vi "Create-romi-sim-model.vi"() -> (2 "Encoder Ft/Count":dbl, 3 "out DiffDriveTrainSim":T1 {"m_Motor"."Jr_KgM2" format="%13.5p"; "m_Motor"."L_H" format="%13.5p"; "m_Motor"."Kt_NMPerAmp" format="%13.5p"; "m_Motor"."KvINV_RadPerSecPerVolt" format="%13.5p"; "m_Motor"."R_Ohms" format="%13.5p"; "m_Motor"."FreeSpeed_RadPerSec" format="%13.5p"; "m_Motor"."FreeCurrent_Amps" format="%13.5p"; "m_Motor"."StallCurrent_Amps" format="%13.5p"; "m_Motor"."StallTorque_NM" format="%13.5p"; "m_Motor"."nominalVoltage_Volts" format="%13.5p"})   [LabVIEW 2020]
uses:
  <vilib>/Rock Robotics/WPI/ThirdParty/JAS_Junk/TrajLib/DIFF_DRIVE_TRAIN_SIM.ctl
  <vilib>/Rock Robotics/WPI/ThirdParty/JAS_Junk/TrajLib/LINEAR_SYSTEM.ctl
  <vilib>/Analysis/Matrix/Datatypes/RealMatrix.ctl
  <vilib>/Rock Robotics/WPI/ThirdParty/JAS_Junk/TrajLib/DCMOTOR.CTL
  <vilib>/Rock Robotics/WPI/ThirdParty/JAS_Junk/TrajLib/DCMOTOR_TYPES_ENUM.ctl
  <vilib>/Rock Robotics/WPI/ThirdParty/JAS_Junk/TrajLib/DCMotor_GetCIM.vi
  <vilib>/Rock Robotics/WPI/ThirdParty/JAS_Junk/TrajLib/DCMotor_GetAndymark9015.vi
  <vilib>/Rock Robotics/WPI/ThirdParty/JAS_Junk/TrajLib/DCMotor_GetAndymarkRs775_125.vi
  <vilib>/Rock Robotics/WPI/ThirdParty/JAS_Junk/TrajLib/DCMotor_GetBag.vi
  <vilib>/Rock Robotics/WPI/ThirdParty/JAS_Junk/TrajLib/DCMotor_GetBanebotsRs550.vi
  <vilib>/Rock Robotics/WPI/ThirdParty/JAS_Junk/TrajLib/DCMotor_GetBanebotsRs775.vi
  <vilib>/Rock Robotics/WPI/ThirdParty/JAS_Junk/TrajLib/DCMotor_GetFalcon500.vi
  <vilib>/Rock Robotics/WPI/ThirdParty/JAS_Junk/TrajLib/DCMotor_GetMiniCIM.vi
  <vilib>/Rock Robotics/WPI/ThirdParty/JAS_Junk/TrajLib/DCMotor_GetNEO.vi
  <vilib>/Rock Robotics/WPI/ThirdParty/JAS_Junk/TrajLib/DCMotor_GetNEO550.vi
  <vilib>/Rock Robotics/WPI/ThirdParty/JAS_Junk/TrajLib/DCMotor_GetRomiBuiltIn.vi
  <vilib>/Rock Robotics/WPI/ThirdParty/JAS_Junk/TrajLib/DCMotor_GetVex775Pro.vi
  <vilib>/Rock Robotics/WPI/ThirdParty/JAS_Junk/TrajLib/LinearSystem_New.vi
  <vilib>/Rock Robotics/WPI/ThirdParty/JAS_Junk/TrajLib/MatBuilder_Create.vi
  <vilib>/Rock Robotics/WPI/ThirdParty/JAS_Junk/TrajLib/MatBuilder_Fill.vi
  <vilib>/Rock Robotics/WPI/ThirdParty/JAS_Junk/TrajLib/MatrixHelper_Zero.vi
  <vilib>/Rock Robotics/WPI/ThirdParty/JAS_Junk/TrajLib/Rotation_CreateAngle.vi
  <vilib>/Rock Robotics/WPI/ThirdParty/JAS_Junk/TrajLib/Translation_Create.vi
  <vilib>/Rock Robotics/WPI/ThirdParty/JAS_Junk/TrajLib/DCMotor_New.vi
  <vilib>/Rock Robotics/WPI/ThirdParty/JAS_Junk/TrajLib/Units_RotationsPerMinuteToRadiansPerSecond.vi
  <vilib>/Rock Robotics/WPI/ThirdParty/JAS_Junk/TrajLib/MatrixHelper_CoerceSize.vi
  <vilib>/Rock Robotics/WPI/ThirdParty/JAS_Junk/TrajLib/Trajectory_Library.lvlib
  <vilib>/Analysis/Matrix/NI_Matrix.lvlib
panel:
  # "<States, 1>"
  # "<Outputs, 1>"
  # "<Inputs, 1>"
  # "<Outputs, 1>"
  # "<States,States>"
  # "<States,Inputs>"
  # "<Outputs,States>"
  # "<Outputs,Inputs>"
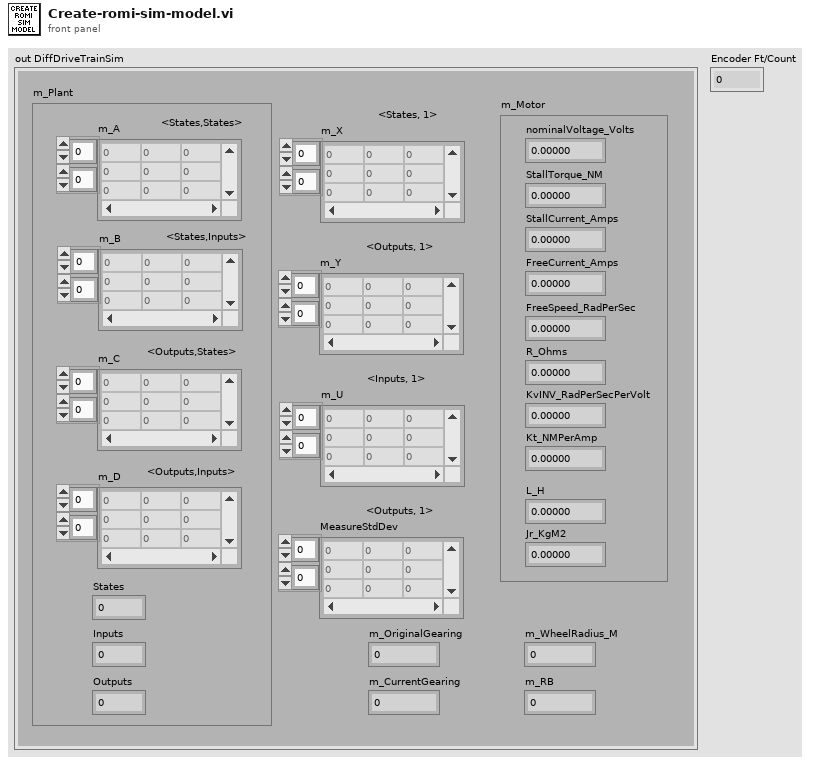
[diagram p1: front panel]
types:
  T1 = typedef "Trajectory_Library.lvlib/DIFF_DRIVE_TRAIN_SIM.ctl" = cluster{"m_Plant":T2, "m_X":T3, "m_Y":T3, "m_U":T3, "MeasureStdDev":T3, "m_Motor":T4, "m_OriginalGearing":dbl, "m_CurrentGearing":dbl, "m_WheelRadius_M":dbl, "m_RB":dbl}
  T2 = typedef "Trajectory_Library.lvlib/LINEAR_SYSTEM.ctl" = cluster{"m_A":T3, "m_B":T3, "m_C":T3, "m_D":T3, "States":i32, "Inputs":i32, "Outputs":i32}
  T3 = typedef "NI_Matrix.lvlib/RealMatrix.ctl" = dbl[][]
  T4 = typedef "Trajectory_Library.lvlib/DCMOTOR.CTL" = cluster{"nominalVoltage_Volts":dbl, "StallTorque_NM":dbl, "StallCurrent_Amps":dbl, "FreeCurrent_Amps":dbl, "FreeSpeed_RadPerSec":dbl, "R_Ohms":dbl, "KvINV_RadPerSecPerVolt":dbl, "Kt_NMPerAmp":dbl, "L_H":dbl, "Jr_KgM2":dbl}
  T5 = typedef "Trajectory_Library.lvlib/DCMOTOR_TYPES_ENUM.ctl" = enum16{"CIM", "AndyMark 9015", "Andy Mark RS 775 125", "Bag", "BaneBots RS 550", "BaneBots RS 775", "Falcon 500", "Mini CIM", "NEO", "NEO 550", "Romi BuiltIn", "Vex 775 Pro"}
  T6 = typedef "Trajectory_Library.lvlib/POSE2D.ctl" = cluster{"TRANSLATION":T7, "ROTATION":T8}
  T7 = typedef "Trajectory_Library.lvlib/TRANSLATION2D.ctl" = cluster{"X":dbl, "Y":dbl}
  T8 = typedef "Trajectory_Library.lvlib/ROTATION2D.ctl" = cluster{"VALUE":dbl, "COS":dbl, "SIN":dbl}
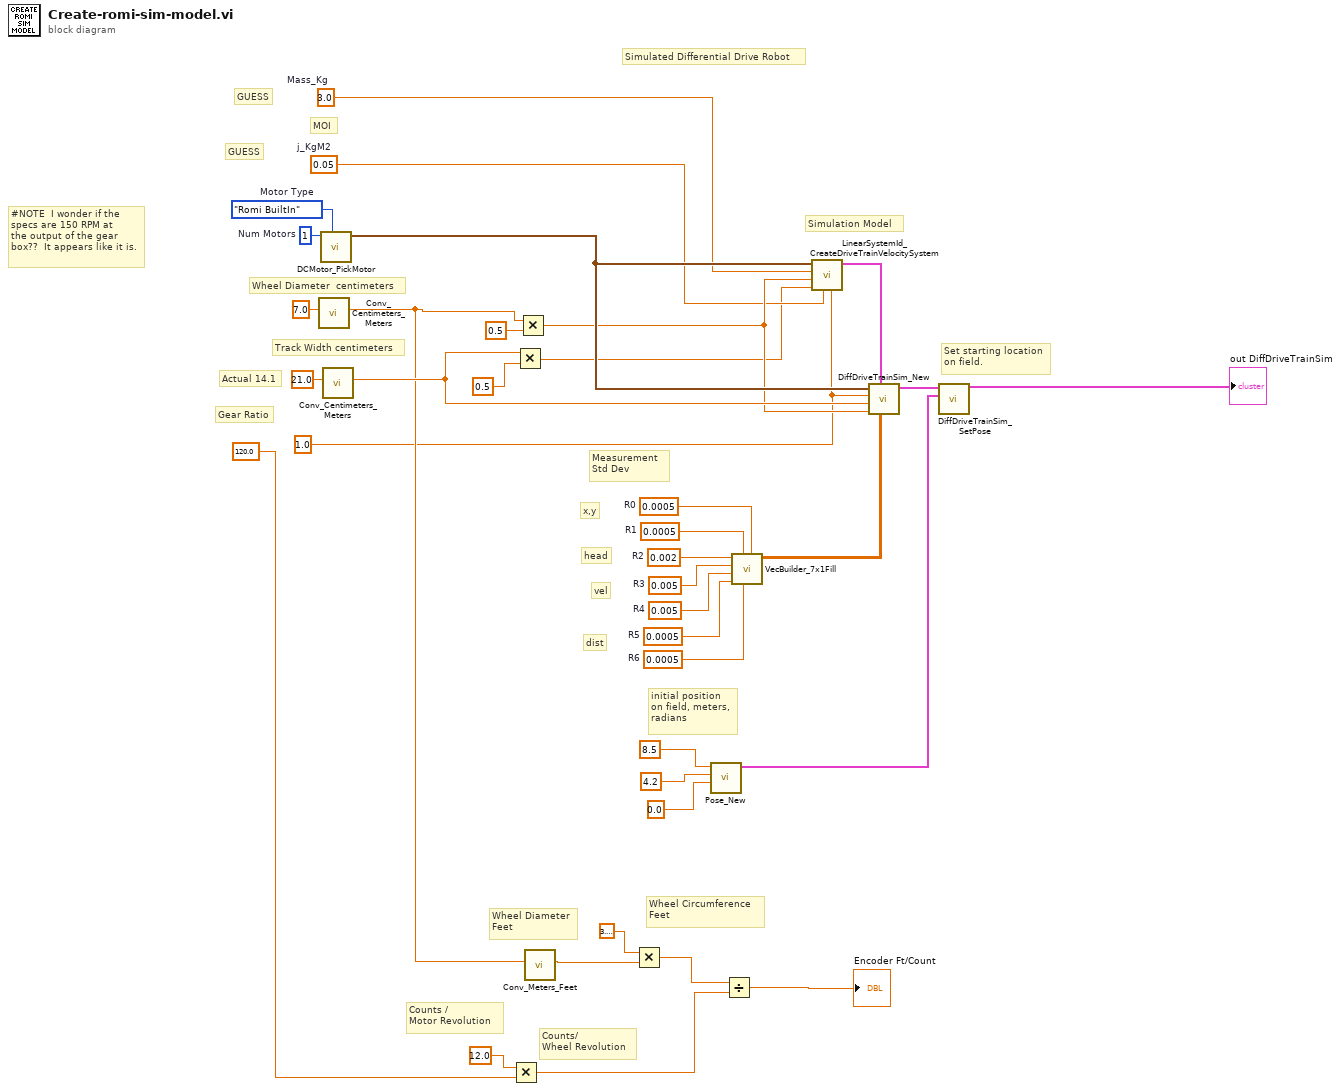
[diagram p0: block diagram]
diagram:
  w1 = 1.0 ("INCH")
  w30 = 1  # Num Motors
  w31 = DCMOTOR_TYPES_ENUM."Romi BuiltIn"  # Motor Type
  w24 = 3.0  # Mass_Kg
  w26 = 0.05  # j_KgM2
  w15 = 0.0005  # R6
  w16 = 0.0005  # R5
  w17 = 0.005  # R4
  w18 = 0.005  # R3
  w19 = 0.002  # R2
  w20 = 0.0005  # R1
  w21 = 0.0005  # R0
  # "Actual 14.1"
  # "#NOTE  I wonder if the \nspecs are 150 RPM at\nthe output of the gear\nbox??  It appears like it is."
  # "Wheel Circumference\nFeet"
  # "Wheel Diameter\nFeet"
  # "Counts/\nWheel Revolution"
  # "Counts /\nMotor Revolution"
  # "Set starting location\non field."
  # "Measurement \nStd Dev"
  # "Gear Ratio"
  # "GUESS"
  # "GUESS"
  # "Track Width centimeters"
  # "Wheel Diameter  centimeters"
  # "MOI"
  # "dist"
  # "vel"
  # "head"
  # "x,y"
  # "Simulated Differential Drive Robot"
  # "initial position\non field, meters,\nradians"
  # "Simulation Model"
  n1 = call <vilib>:"Conv_Centimeters_Meters.vi"("Centimeter"=7.0 ("INCH")) -> ("Meters"=w8:dbl)  [unwired: 10 in]
  n2 = call <vilib>:"DCMotor_PickMotor.vi"("DCMOTOR_TYPES"=w31, "Num Motors"=w30) -> ("DCMOTOR"=w32:T4)  [unwired: 9 in]
  n3 = call <vilib>:"Conv_Centimeters_Meters.vi"("Centimeter"=21.0 ("INCH")) -> ("Meters"=w33:dbl)  [unwired: 10 in]
  n4 = Multiply(x=12.0, y=120.0 ("INCH")) -> (x*y=w7:dbl)
  n5 = Multiply(x=w33, y=0.5) -> (x*y=w25:dbl)
  n6 = Multiply(x=w8, y=0.5) -> (x*y=w27:dbl)
  n7 = call <vilib>:"Conv_Meters_Feet.vi"("Meters"=w8) -> ("Feet"=w5:dbl)  [unwired: 10 in]
  n8 = Multiply(x=3.141592653589793, y=w5) -> (x*y=w4:dbl)
  n9 = call <vilib>:"Pose_New.vi"("Heading"=0.0, "Y"=4.2, "X"=8.5) -> ("out POSe"=w14:T6)  [unwired: 8 in]
  n10 = Divide(x=w4, y=w7) -> (x/y=→"Encoder Ft/Count":dbl)
  n11 = call <vilib>:"VecBuilder_7x1Fill.vi"("R0"=w21, "R6"=w15, "R1"=w20, "R5"=w16, "R4"=w17, "R3"=w18, "R2"=w19) -> ("output matrix"=w35:T3)  [unwired: 4 in]
  n12 = call <vilib>:"LinearSystemId_CreateDriveTrainVelocitySystem.vi"("G"=w1, "JKgMetersSquared"=w26, "rbMeters"=w25, "rMeters"=w27, "MassKg"=w24, "Motor"=w32) -> ("Linearsystem"=w23:T2)  [unwired: 4 in, 1 out]
  n13 = call <vilib>:"DiffDriveTrainSim_New.vi"("MeasurementStdDev"=w35, "DriveTrainPlant"=w23, "WheelRadius_M"=w27, "TrackWidth_M"=w33, "Gearing"=w1, "DriveMotor"=w32) -> ("DiffDriveTrainSim"=w36:T1)  [unwired: 5 in]
  n14 = call <vilib>:"DiffDriveTrainSim_SetPose.vi"("Pose"=w14, "in DiffDriveTrainSim"=w36) -> ("out DiffDriveTrainSim"=→"out DiffDriveTrainSim":T1)  [unwired: 9 in]
